vi "Get Point.vi"(0 "Experiment3D in":refnum<class "Experiment3D.lvclass">, 11 "error in (no error)":errorcluster) -> (4 "Experiment3D out":refnum<class "Experiment3D.lvclass">, 6 "x":dbl, 8 "y":dbl, 10 "z":dbl, 15 "error out":errorcluster)   [LabVIEW 2014, in "Experiment3D.lvclass"]
uses:
  Experiment3D.lvclass
  Data/Data3D/Data3D.lvclass
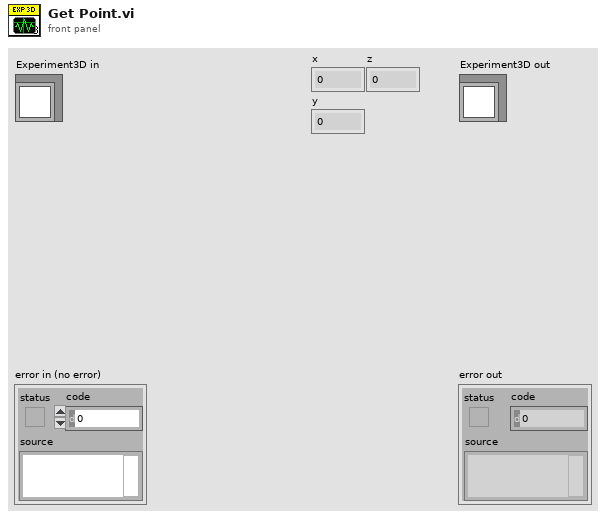
[diagram p1: front panel]
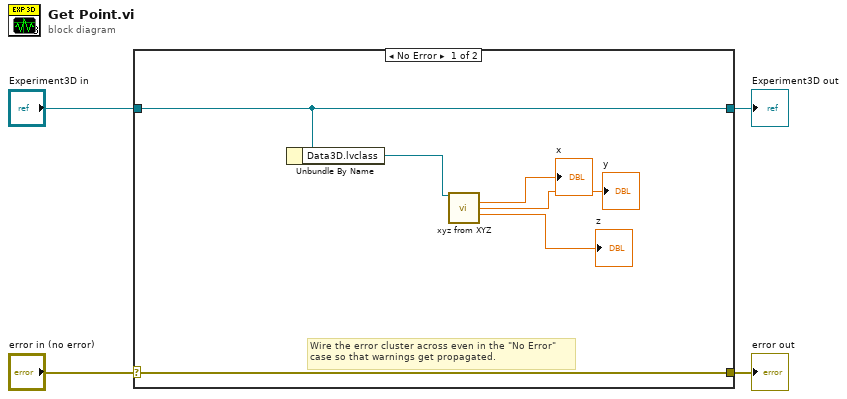
[diagram p0: block diagram]
diagram:
  n1 = case shown="No Error" "error in (no error)" {
    selector: "error in (no error)" -> [w10 w12]
    tunnel: [w10 w12] -> w3
    tunnel: [w9 w11] -> w1
    tunnel: "Experiment3D in" -> [w9 w11]
    frame No Error {
      # "Wire the error cluster across even in the \"No Error\"\ncase so that warnings get propagated."
      n2 = Unbundle By Name(w9) -> ("Data3D.lvclass"=w8:refnum<class "Data3D.lvclass">)
      n3 = call "xyz from XYZ.vi"("Data3D in"=w8) -> ("x"=→"x":dbl, "y"=→"y":dbl, "z"=→"z":dbl)  [unwired: 10 in, 2 out]
    }
    frame Error {
    }
  }
  "error out" <- w3
  "Experiment3D out" <- w1
